vi "convert error list.vi"   [LabVIEW 2020]
uses:
  Error Description.ctl
types:
  T1 = cluster{"Description":string, "Details":string}[]
  T2 = typedef "Error Description.ctl" = cluster{"Code":i32, "Description":string, "Details":string}
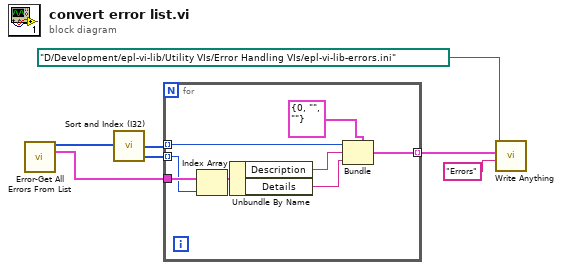
[diagram p0: block diagram]
diagram:
  n1 = call "Error-Get All Errors From List.vi"() -> ("Codes"=w3:i32[], "Errors"=w7:T1)  [unwired: 12 in, 2 out]
  n2 = call "Sort and Index (I32).vi"("X"=w3) -> ("Index"=w1:i32[], "Sort(X)"=w2:i32[])  [unwired: 3 in]
  n3 = for {
    tunnel: w2 -> [w14] mode=indexing
    tunnel: w7 -> [w15]
    tunnel: [w11] -> w4 mode=indexing
    tunnel: w1 -> [w8] mode=indexing
    n4 = Index Array(array=w15, index=w8) -> (element=w9:cluster{"Description":string, "Details":string})
    n5 = Unbundle By Name(w9) -> ("Description"=w13:string, "Details"=w12:string)
    n6 = Bundle(cluster=T2 {"Code"=0, "Description"="", "Details"=""} ("error"), "Code"=w14, "Description"=w13, "Details"=w12) -> (w11:T2)
  }
  n7 = call "Write Anything.vi"("Section Name (Name of \"Anything\")"="Errors" ("Section Name (Name of \"Anything\")"), "Anything"=w4, "Path (dialog)"=path "D:/Development/epl-vi-lib/Utility VIs/Error Handling VIs/epl-vi-lib-errors.ini") -> ()  [unwired: 7 in, 2 out]
